vi "Test Base Main.vi"() -> ()   [LabVIEW 2013]
doc: "This Continuous Measurement sample project is based on the Queued Message Handler template.\n\nThe Event Handling Loop generates messages based on user interface actions.\n\nThe Message Handling Loop processes messages generated by the Event Handling Loop, or by other messages. There are also Acquisition and Logging message handling loop subVIs, and a chart updating loop."
uses:
  Settings/Settings.ctl
  Acquisition/Hardware Configuration.ctl
  Acquisition/Signal Type.ctl
  Logging/Logging Configuration.ctl
  controls/UI Data.ctl
  controls/UI State.ctl
  <vilib>/Utility/error.llb/DialogType.ctl
  support/Message Queue/Message Cluster.ctl
  support/Message Queue/Enqueue Message (Single).vi
  <vilib>/Utility/error.llb/Error Cluster From Error Code.vi
  <vilib>/ErrorRing/Error Ring.xnode
  Acquisition/Acquisition.lvlib
  Logging/Logging.lvlib
  Settings/Settings.lvlib
  support/User Event - Stop/User Event - Stop.lvlib
  support/Message Queue/Message Queue.lvlib
  support/Message Queue/Enqueue Message (MultiLine String w Array).vi
panel:
  in  "Test Logging Error Handler":bool
  in  "Test Acquisition Error Handler":bool
  out "Data":waveform(dbl)[](graph)
  in  "Settings":bool
  in  "Start":bool
  in  "Stop":bool
  out "Status":string
  in  "Exit":bool
  # "Continuous Measurement Data Logger"
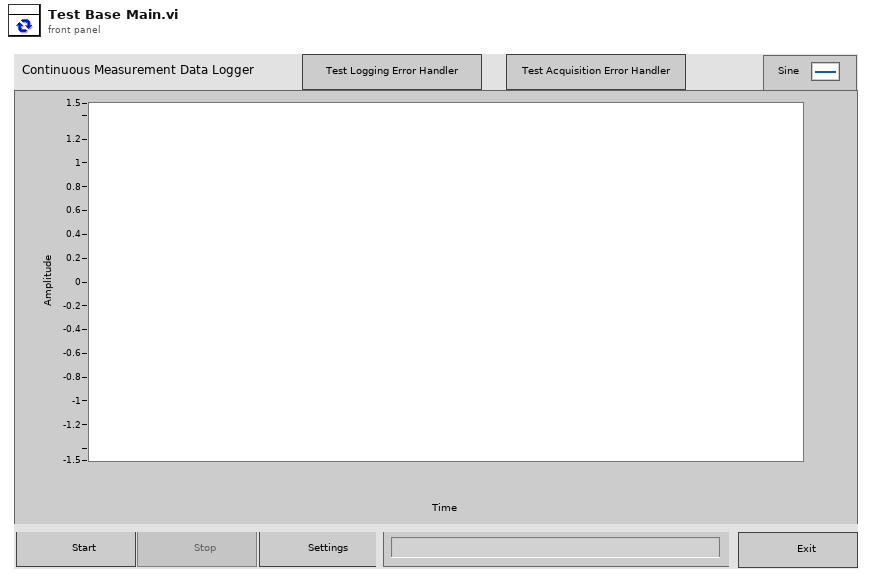
[diagram p1: front panel]
types:
  T1 = cluster{"Macro:Initialize":string, "Macro:Exit":string, "Core":cluster{"Current VI Reference":refnum<vi>, "Close Panel on Exit?":bool}}
  T2 = typedef "UI State.ctl" = enum16{"Idle", "Acquiring and Logging", "Waiting for Exit", "Waiting for Exit (Acq Stopped)", "Waiting for Exit (Log Stopped)", "Waiting for Stop", "Waiting for Stop (Acq Stopped)", "Waiting for Stop (Log Stopped)"}
  T3 = typedef "UI Data.ctl" = cluster{"Start Ref":refnum<vi>, "Stop Ref":refnum<vi>, "Settings Ref":refnum<vi>, "Exit Ref":refnum<vi>, "Status Ref":refnum<vi>, "Data Ref":refnum<vi>}
  T4 = typedef "Settings.lvlib/Settings.ctl" = cluster{"Hardware Configuration":T5, "Logging Configuration":T7}
  T5 = typedef "Acquisition.lvlib/Hardware Configuration.ctl" = cluster{"HW Refnum <Replace Me>":string, "Signal Type <Replace Me>":T6}
  T6 = typedef "Acquisition.lvlib/Signal Type.ctl" = enum16{"Sine Wave", "Square with Noise"}
  T7 = typedef "Logging.lvlib/Logging Configuration.ctl" = cluster{"Log File Base Path":path, "TDMS File Reference":refnum<k34>}
  T8 = typedef "Message Queue.lvlib/All Message Queues.ctl" = cluster{"UI":refnum<queue>, "Acquisition":refnum<queue>, "Logging":refnum<queue>}
  T9 = enum32{"invalid app kind", "Development System", "Run Time System", "Student Edition", "Embedded LabVIEW", "Evaluation", "Custom"}
  T10 = typedef "Message Queue.lvlib/Message Cluster.ctl" = cluster{"Message":string, "Message Data":variant}
  T11 = enum32{"Invalid", "Standard", "Closed", "Hidden", "Minimized", "Maximized"}
  T12 = typedef "DialogType.ctl" = u16
  T13 = cluster{"element":T10, "error constant":errorcluster}
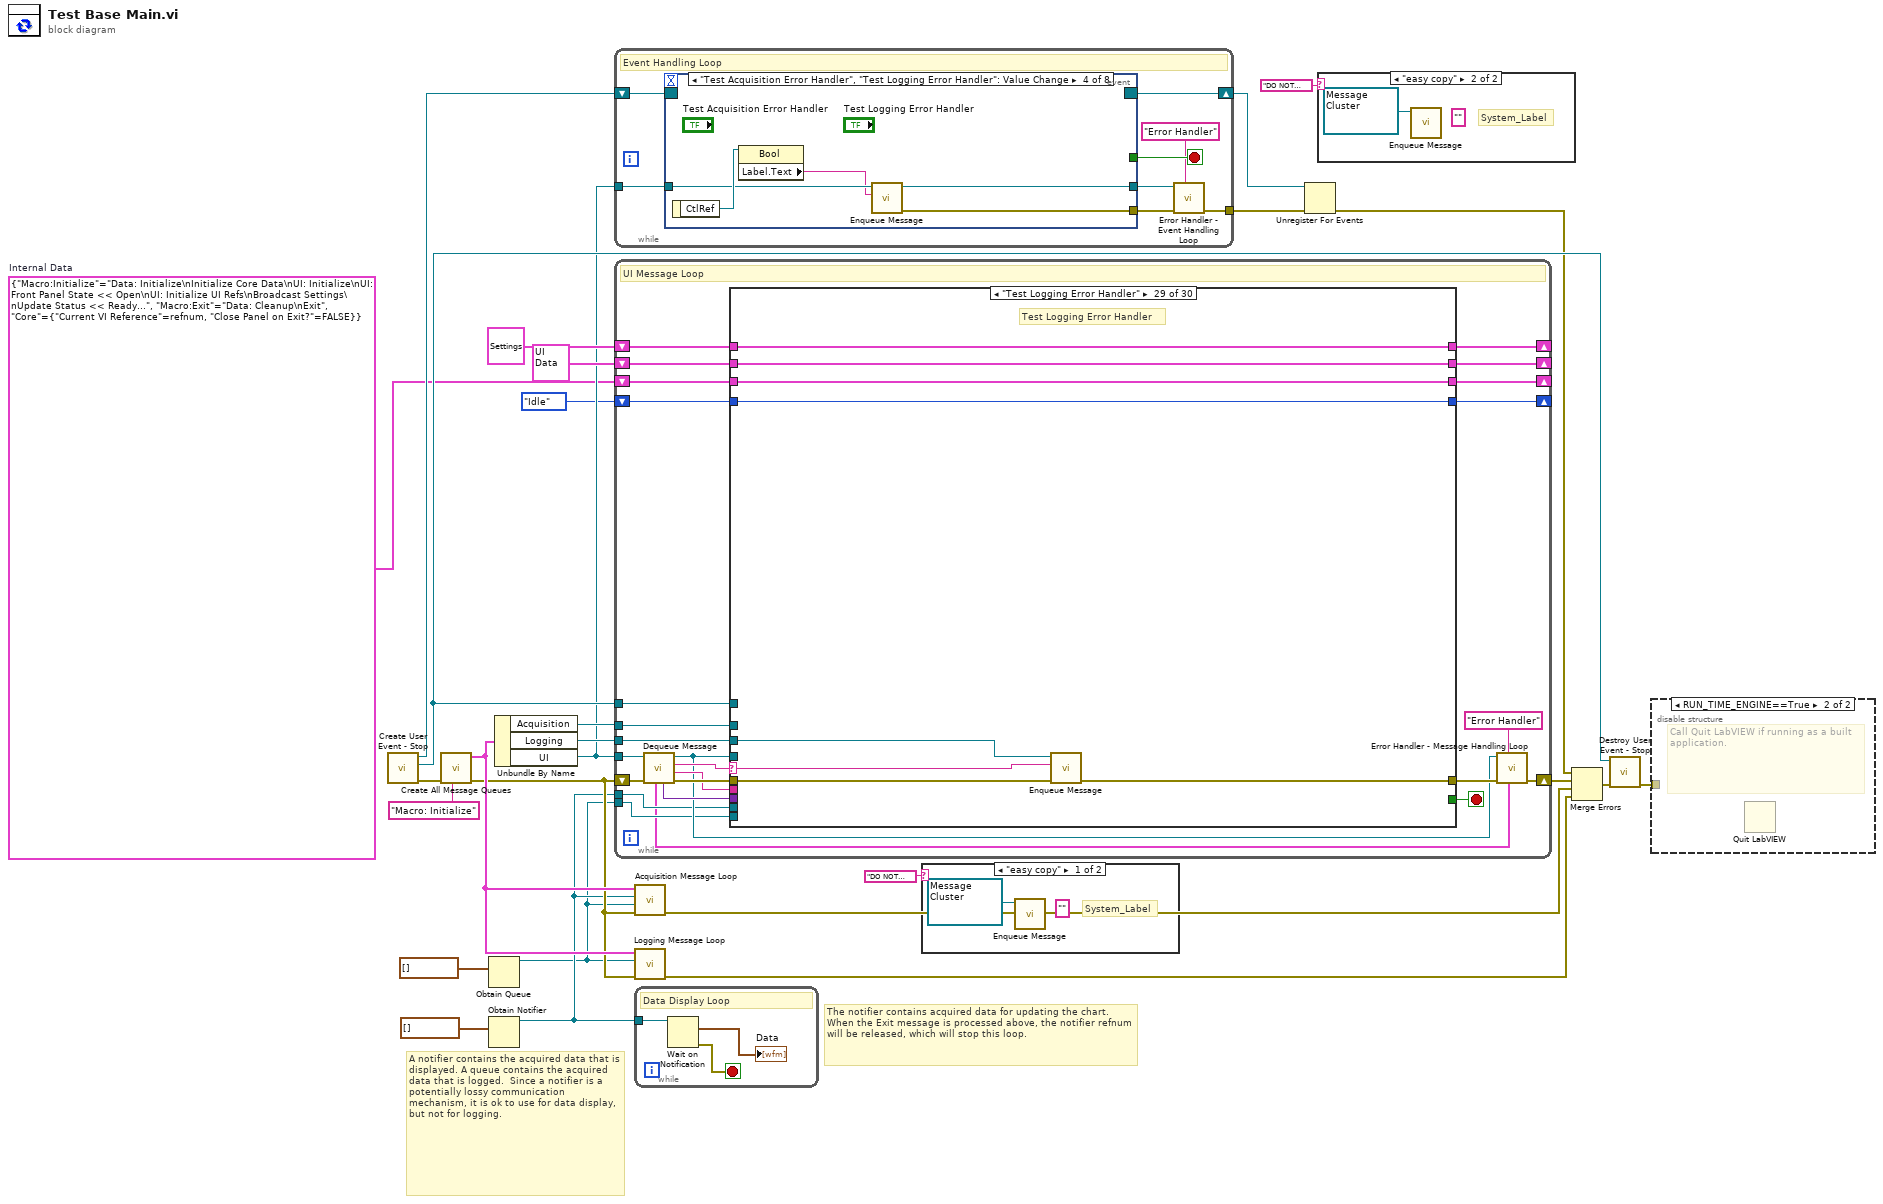
[diagram p0: block diagram]
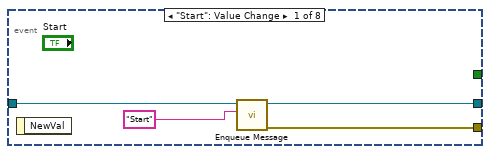
[diagram p5: hidden frame]
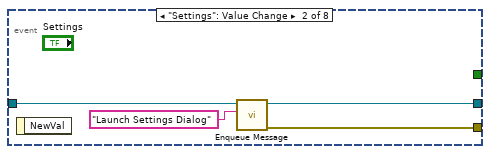
[diagram p6: hidden frame]
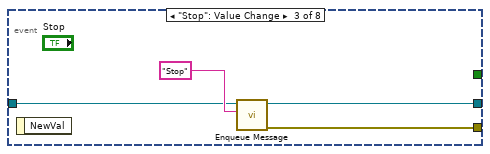
[diagram p7: hidden frame]
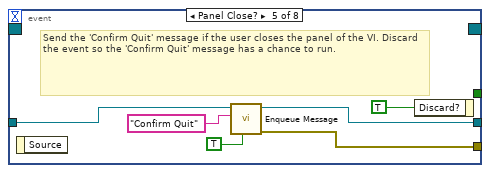
[diagram p8: hidden frame]
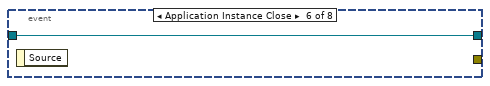
[diagram p9: hidden frame]
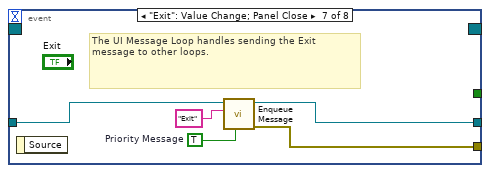
[diagram p10: hidden frame]
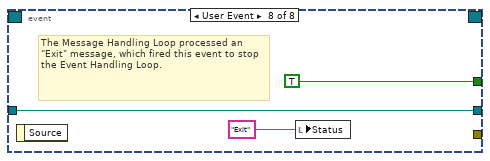
[diagram p11: hidden frame]
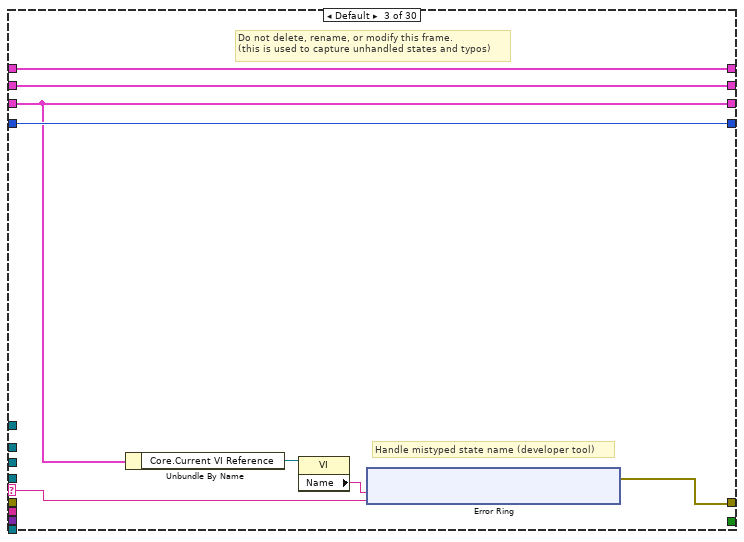
[diagram p14: hidden frame]
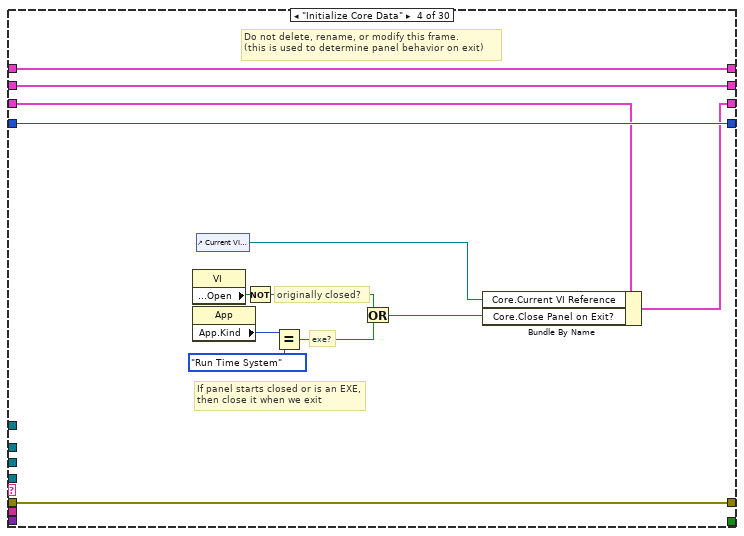
[diagram p15: hidden frame]
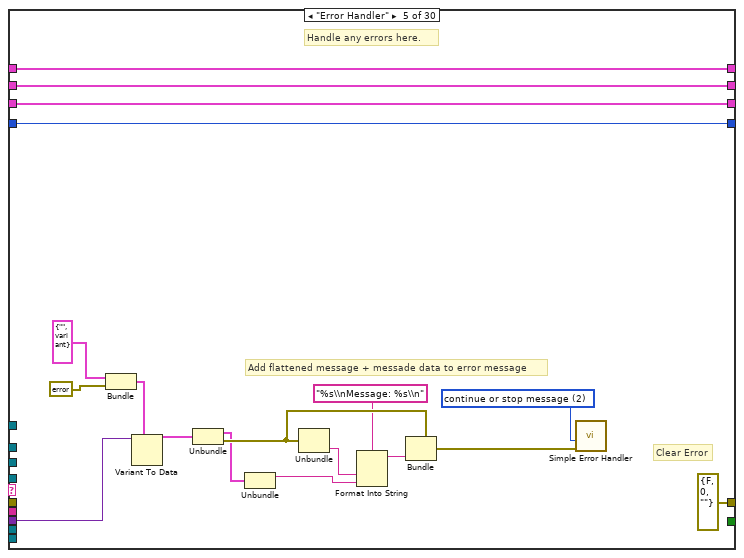
[diagram p16: hidden frame]
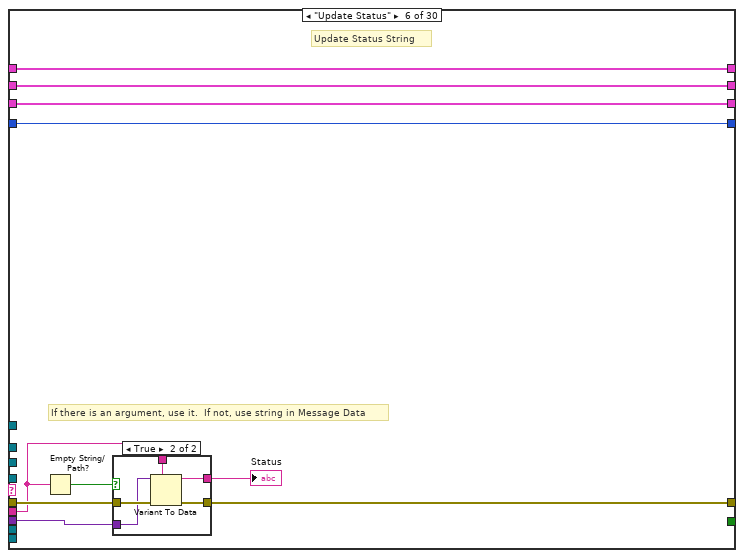
[diagram p17: hidden frame]
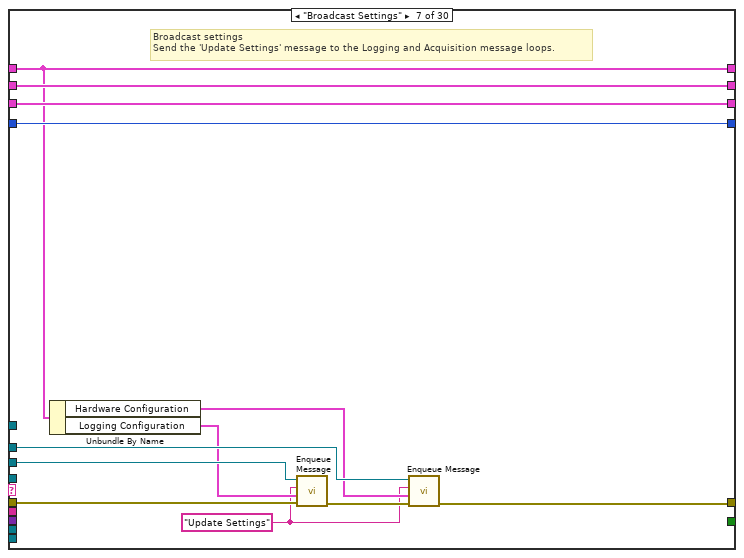
[diagram p19: hidden frame]
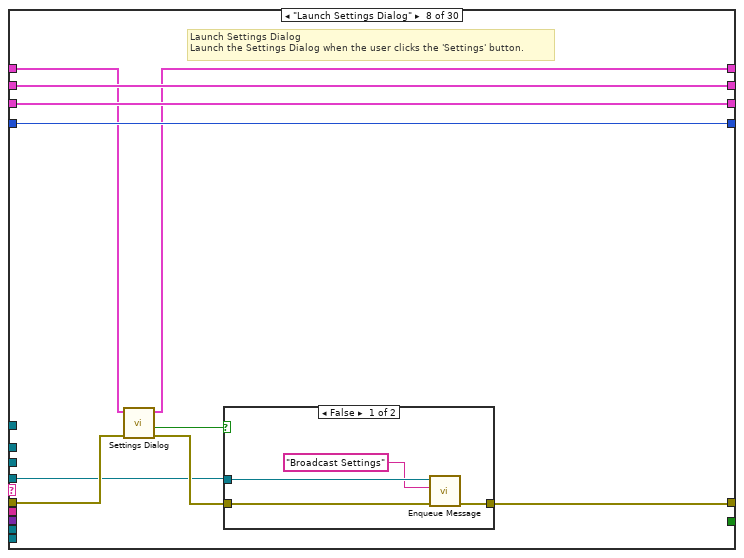
[diagram p20: hidden frame]
diagram:
  w4 = T1 {"Macro:Initialize"="Data: Initialize\nInitialize Core Data\nUI: Initialize\nUI: Front Panel State << Open\nUI: Initialize UI Refs\nBroadcast Settings\nUpdate Status << Ready...", "Macro:Exit"="Data: Cleanup\nExit", "Core"={"Current VI Reference"=refnum, "Close Panel on Exit?"=FALSE}}  # Internal Data
  # "A notifier contains the acquired data that is displayed. A queue contains the acquired data that is logged.  Since a notifier is a potentially lossy communication mechanism, it is ok to use for data display, but not for logging."
  # "The notifier contains acquired data for updating the chart. When the Exit message is processed above, the notifier refnum will be released, which will stop this loop."
  n1 = call "Create User Event - Stop.vi"() -> ("error out"=w22:errorcluster, "User Event - Stop"=w24:refnum<user-event>, "Stop Event Registration Refnum"=w25:refnum<event-registration>)  [unwired: 9 in]
  n2 = call "Create All Message Queues.vi"("Message"="Macro: Initialize", "error in (no error)"=w22) -> ("error out"=w19:errorcluster, "Message Queues out"=w21:T8)  [unwired: 8 in]
  n3 = Obtain Queue(element data type=waveform(dbl)[] []) -> (queue out=w8:refnum<queue>)  [unwired: 4 in, 2 out]
  n4 = Obtain Notifier(notification data type=waveform(dbl)[] []) -> (notifier out=w10:refnum<notifier>)  [unwired: 3 in, 2 out]
  n5 = Unbundle By Name(w21) -> ("Acquisition"=w14:refnum<queue>, "Logging"=w13:refnum<queue>, "UI"=w12:refnum<queue>)
  n6 = while {
    tunnel: w12 -> [w34]
    tunnel: [w31] -> w26
    shift-right: [w33] -> w16
    shift-left: w25 -> [w35]
    stop <- w32 stop-if-true
    # "Event Handling Loop"
    n7 = event shown="[3] \"Test Acquisition Error Handler\", \"Test Logging Error Handler\": Value Change" {
      selector: w35 -> [_ _ _ _ _ _ _ _]
      dyn-events: [_ _ _ _ _ _ _ _] -> w33
      timeout: _ -> [_ _ _ _ _ _ _ _]
      tunnel: [_ _ _ _ _ _ _ TRUE ("Discard?")] -> w32
      tunnel: w34 -> [w39 w41 w46 w51 w56 w59 w61 w65]
      tunnel: [w37 w43 w45 w49 w54 _ w64 _] -> w30
      tunnel: [w36 w40 w44 w50 w55 w59 w60 w65] -> w29
      event "Start": Value Change {
        n8 = event-data() -> ()  [unwired: 1 in, 1 out]
        n9 = call-poly "Enqueue Message.vi"("Message"="Start", "Message Queue"=w39) -> ("error out"=w37:errorcluster, "dup Message Queue"=w36:refnum<queue>)  [unwired: 8 in]
      }
      event "Settings": Value Change {
        n10 = event-data() -> ()  [unwired: 1 in, 1 out]
        n11 = call-poly "Enqueue Message.vi"("Message"="Launch Settings Dialog", "Message Queue"=w41) -> ("error out"=w43:errorcluster, "dup Message Queue"=w40:refnum<queue>)  [unwired: 8 in]
      }
      event "Stop": Value Change {
        n12 = event-data() -> ()  [unwired: 1 in, 1 out]
        n13 = call-poly "Enqueue Message.vi"("Message"="Stop", "Message Queue"=w46) -> ("error out"=w45:errorcluster, "dup Message Queue"=w44:refnum<queue>)  [unwired: 8 in]
      }
      event "Test Acquisition Error Handler", "Test Logging Error Handler": Value Change {
        n14 = event-data() -> ("CtlRef"=w52:refnum<vi>)  [unwired: 1 in]
        n15 = property class="Bool"(reference=w52) -> ("Label.Text"=w48:string)  [unwired: 1 in, 2 out]
        n16 = call-poly "Enqueue Message.vi"("Message"=w48, "Message Queue"=w51) -> ("error out"=w49:errorcluster, "dup Message Queue"=w50:refnum<queue>)  [unwired: 8 in]
      }
      event Panel Close? {
        # "Send the 'Confirm Quit' message if the user closes the panel of the VI. Discard the event so the 'Confirm Quit' message has a chance to run."
        n17 = event-data() -> ()  [unwired: 1 in, 1 out]
        n18 = call-poly "Enqueue Message.vi"("Priority Message? (F)"=TRUE, "Message"="Confirm Quit", "Message Queue"=w56) -> ("error out"=w54:errorcluster, "dup Message Queue"=w55:refnum<queue>)  [unwired: 7 in]
        n19 = event-data("Discard?"=TRUE) -> ()  [unwired: 1 in, 1 out]
      }
      event Application Instance Close {
        n20 = event-data() -> ()  [unwired: 1 in, 1 out]
      }
      event "Exit": Value Change; Panel Close {
        w62 = TRUE  # Priority Message
        # "The UI Message Loop handles sending the Exit message to other loops."
        n21 = event-data() -> ()  [unwired: 1 in, 1 out]
        n22 = call-poly "Enqueue Message.vi"("Priority Message? (F)"=w62, "Message"="Exit", "Message Queue"=w61) -> ("error out"=w64:errorcluster, "dup Message Queue"=w60:refnum<queue>)  [unwired: 7 in]
      }
      event User Event {
        # "The Message Handling Loop processed an \"Exit\" message, which fired this event to stop the Event Handling Loop."
        n23 = event-data() -> ()  [unwired: 1 in, 1 out]
        n24 = local write "Status"("Exit" ("Exit String")) -> ()
      }
    }
    n25 = call "Error Handler - Event Handling Loop.vi"("Error Handler Message"="Error Handler" ("Message"), "error in (no error)"=w30, "Message Queue"=w29) -> ("dup error in"=w31:errorcluster)  [unwired: 7 in, 1 out]
  }
  n26 = while {
    tunnel: w12 -> [w91]
    tunnel: w24 -> [w87]
    shift-right: [w90] -> w27
    shift-left: w19 -> [w92]
    shift-right: [w78] -> _
    shift-left: T4 {"Hardware Configuration"={"HW Refnum <Replace Me>"="", "Signal Type <Replace Me>"=enum."Sine Wave"}, "Logging Configuration"={"Log File Base Path"=path "", "TDMS File Reference"=refnum}} ("Settings") -> [w80]
    shift-right: [w77] -> _
    shift-left: T3 {"Start Ref"=refnum, "Stop Ref"=refnum, "Settings Ref"=refnum, "Exit Ref"=refnum, "Status Ref"=refnum, "Data Ref"=refnum} ("Measurement UI Controls") -> [w79]
    tunnel: w14 -> [w86]
    tunnel: w13 -> [w85]
    tunnel: w10 -> [w70]
    tunnel: w8 -> [w69]
    shift-right: [w84] -> _
    shift-left: UI_State."Idle" ("UI State") -> [w83]
    shift-right: [w73] -> _
    shift-left: w4 -> [w74]
    stop <- w82 stop-if-true
    # "UI Message Loop"
    n27 = call "Dequeue Message.vi"("error in (no error)"=w92, "Message Queue"=w91) -> ("error out"=w89:errorcluster, "Argument"=w76:string, "Message"=w88:string, "dup Message Queue"=w72:refnum<queue>, "Message Data"=w75:variant, "element"=w68:T10)  [unwired: 4 in]
    n28 = case shown="\"Test Logging Error Handler\"" w88 {
      selector: w88 -> [_ _ w104 _ _ _ _ _ _ _ _ _ _ _ _ _ _ _ _ _ w346 _ _ _ _ _ _ w471 w480 _]
      tunnel: w79 -> [w96 w100 w109 w123 w149 w158 w178 w188 w201 w238 w243 w252 w255 w262 w267 w279 w292 w303 w333 w342 w361 w367 w388 w408 w418 w444 w467 w476 w484 w488]
      tunnel: w76 -> [_ _ _ _ _ w151 _ _ _ _ _ _ _ _ _ _ w293 w304 _ _ _ _ _ _ _ _ _ _ _ _]
      tunnel: w80 -> [w95 w101 w110 w121 w147 w159 w171 w185 w195 w240 w244 w250 w256 w263 w269 w289 w296 w306 w334 w343 w359 w368 w390 w410 w420 w446 w468 w477 w485 w489]
      tunnel: [w97 w102 w103 w131 errorcluster {"status"=FALSE, "code"=0, "source"=""} ("error out") w153 w167 w179 w194 w230 w245 w248 w257 w264 w268 w288 w294 w307 w335 w338 w348 w369 w371 w391 w415 w439 w469 w470 w479 w490] -> w81
      tunnel: w89 -> [w97 w102 _ w131 _ w155 w175 w183 w198 w228 w245 w249 w258 w264 w268 w288 w295 w308 w335 w340 w358 w369 w378 w393 w416 w440 w469 w473 w481 w490]
      tunnel: [w96 w100 w109 w123 w149 w158 w178 w188 w201 w238 w243 w252 w255 w262 w267 w270 w292 w303 w333 w342 w361 w367 w388 w408 w418 w444 w467 w476 w484 w488] -> w77
      tunnel: [_ _ _ _ _ _ _ _ _ TRUE _ _ _ _ _ _ _ _ _ _ _ _ _ _ _ _ _ _ _ _] -> w82
      tunnel: [w95 w101 w110 w121 w147 w159 w171 w184 w195 w240 w244 w247 w256 w263 w269 w289 w296 w306 w334 w343 w359 w368 w390 w410 w420 w446 w468 w477 w485 w489] -> w78
      tunnel: w87 -> [_ _ _ _ _ _ _ _ _ w229 _ _ _ _ _ _ _ _ _ _ _ _ _ _ _ _ _ _ _ _]
      tunnel: w86 -> [_ _ _ _ _ _ w172 _ _ w227 _ _ _ _ _ _ _ _ _ _ w344 _ w373 w398 _ _ _ w472 _ _]
      tunnel: w85 -> [_ _ _ _ _ _ w174 _ _ w226 _ _ _ _ _ _ _ _ _ _ w345 _ w375 w399 _ _ _ _ w478 _]
      tunnel: [w94 w99 w108 w122 w148 w157 w177 w187 w196 UI_State."Idle" ("UI State") w242 w251 w254 w261 w266 w287 w291 w302 w332 w341 w360 w366 UI_State."Acquiring and Logging" ("UI State") w394 w414 w442 w466 w475 w483 w487] -> w84
      tunnel: w83 -> [w94 w99 w108 w122 w148 w157 w177 w187 w197 _ w242 w251 w254 w261 w266 w287 w291 w302 w332 w341 w360 w366 _ w395 w413 w443 w466 w475 w483 w487]
      tunnel: w75 -> [_ _ _ _ w132 w154 _ _ _ _ _ _ _ _ _ _ _ _ _ _ _ _ _ _ _ _ _ _ _ _]
      tunnel: w74 -> [w93 w98 w106 w120 w146 w156 w176 w186 w200 w237 w241 w246 w253 w260 w265 w286 w290 w301 w331 w336 w352 w365 w389 w409 w419 w445 w465 w474 w482 w486]
      tunnel: [w93 w98 w106 w119 w146 w156 w176 w186 w200 w237 w241 w246 w253 w260 w265 w286 w290 w301 w331 w336 w352 w365 w389 w409 w419 w445 w465 w474 w482 w486] -> w73
      tunnel: w72 -> [_ _ _ _ _ _ _ w180 w199 w225 _ _ _ _ _ _ _ _ _ w339 w357 _ w377 _ w417 w441 _ _ _ _]
      tunnel: w70 -> [_ _ _ _ _ _ _ _ _ w224 _ _ _ _ _ _ _ _ _ _ _ _ _ _ _ _ _ _ _ _]
      tunnel: w69 -> [_ _ _ _ _ _ _ _ _ w223 _ _ _ _ _ _ _ _ _ _ _ _ _ _ _ _ _ _ _ _]
      frame "", "Idle" {
        # "Executes when the state queue is empty\nAlso commented out messages"
      }
      frame "---------- Core ----------" {
        # "Do not put any code in this frame.\n(it is a separator no-op)"
      }
      frame Default {
        # "Handle mistyped state name (developer tool)"
        # "Do not delete, rename, or modify this frame.\n(this is used to capture unhandled states and typos)"
        n29 = Unbundle By Name(w106) -> ("Core.Current VI Reference"=w105:refnum<vi>)
        n30 = property class="VI"(reference=w105) -> ("Name"=w107:string)  [unwired: 1 in, 2 out]
        n31 = xnode "Error Ring"("parameter 0"=w107, "parameter 1"=w104) -> ("error out"=w103:errorcluster)
      }
      frame "Initialize Core Data" {
        # "Do not delete, rename, or modify this frame.\n(this is used to determine panel behavior on exit)"
        # "originally closed?"
        # "exe?"
        # "If panel starts closed or is an EXE, then close it when we exit"
        n32 = property class="VI"() -> ("Front Panel.Open"=w130:bool)  [unwired: 2 in, 2 out]
        n33 = property class="App"() -> ("App.Kind"=w129:T9)  [unwired: 2 in, 2 out]
        n34 = control-ref of="Current VI Reference"() -> (w124:refnum<vi>)
        n35 = Not(x=w130) -> (.not. x?=w127:bool)
        n36 = Equal?(x=w129, y=T9."Run Time System" ("Application:Kind")) -> (x = y?=w126:bool)
        n37 = Or(x=w127, y=w126) -> (x .or. y?=w125:bool)
        n38 = Bundle By Name(cluster=w120, "Core.Current VI Reference"=w124, "Core.Close Panel on Exit?"=w125) -> (w119:T1)
      }
      frame "Error Handler" {
        w144 = T12 2 items=["no dialog", "OK message", "continue or stop message", "OK message + warnings", "continue/stop + warnings"] ("type of dialog (OK msg:1)")
        # "Add flattened message + messade data to error message"
        # "Clear Error"
        # "Handle any errors here."
        n39 = Bundle("element"=T10 {"Message"="", "Message Data"=variant}, "error constant"=errorcluster {"status"=FALSE, "code"=0, "source"=""}) -> (w141:T13)  [unwired: 1 in]
        n40 = Variant To Data(type=w141, Variant=w132) -> (data=w140:T13)  [unwired: 1 in, 1 out]
        n41 = Unbundle(w140) -> ("element"=w137:T10, "error constant"=w139:errorcluster)
        n42 = Unbundle(w137) -> ("Message"=w135:string)  [unwired: 1 out]
        n43 = Unbundle(w139) -> ("source"=w134:string)  [unwired: 2 out]
        n44 = Format Into String(format string="%s\\nMessage: %s\\n", w134, w135) -> (resulting string=w136:string)  [unwired: 2 in, 1 out]
        n45 = Bundle(cluster=w139, "source"=w136) -> (w138:errorcluster)  [unwired: 2 in]
        n46 = call <vilib>:"Simple Error Handler.vi"("type of dialog (OK msg:1)"=w144, "error in (no error)"=w138) -> ()  [unwired: 3 in, 5 out]
      }
      frame "Update Status" {
        # "If there is an argument, use it.  If not, use string in Message Data"
        # "Update Status String"
        n47 = Empty String/Path?(string/path=w151) -> (empty?=w152:bool)
        n48 = case shown="True" w152 {
          tunnel: w155 -> [w160 w166]
          tunnel: w154 -> [_ w165]
          tunnel: w151 -> [w161 w164]
          tunnel: [w160 w163] -> w153
          tunnel: [w161 w162] -> w150
          frame False {
          }
          frame True {
            n49 = Variant To Data(error in=w166, type=w164, Variant=w165) -> (data=w162:string, error out=w163:errorcluster)
          }
        }
        "Status" <- w150
      }
      frame "Broadcast Settings" {
        w168 = "Update Settings" ("Message")
        # "Broadcast settings\nSend the 'Update Settings' message to the Logging and Acquisition message loops."
        n50 = Unbundle By Name(w171) -> ("Hardware Configuration"=w169:T5, "Logging Configuration"=w170:T7)
        n51 = call-poly "Enqueue Message.vi"("error in (no error)"=w175, "Message Data"=w170, "Message"=w168, "Message Queue"=w174) -> ("error out"=w173:errorcluster)  [unwired: 6 in, 1 out]
        n52 = call-poly "Enqueue Message.vi"("error in (no error)"=w173, "Message Data"=w169, "Message"=w168, "Message Queue"=w172) -> ("error out"=w167:errorcluster)  [unwired: 6 in, 1 out]
      }
      frame "Launch Settings Dialog" {
        # "Launch Settings Dialog\nLaunch the Settings Dialog when the user clicks the 'Settings' button."
        n53 = call "Settings Dialog.vi"("error in (no error)"=w183, "Settings in"=w185) -> ("error out"=w181:errorcluster, "Cancelled?"=w182:bool, "Settings out"=w184:T4)  [unwired: 6 in, 1 out]
        n54 = case shown="False" w182 {
          tunnel: w180 -> [w192 _]
          tunnel: w181 -> [w191 w193]
          tunnel: [w190 w193] -> w179
          frame False {
            n55 = call-poly "Enqueue Message.vi"("error in (no error)"=w191, "Message"="Broadcast Settings", "Message Queue"=w192) -> ("error out"=w190:errorcluster)  [unwired: 7 in, 1 out]
          }
          frame True {
          }
        }
      }
      frame "Confirm Quit" {
        # "Confirm Quit\nMessage that can confirm whether or not the user wants to exit the application."
        n56 = case shown="\"Acquiring and Logging\"" w197 {
          tunnel: w199 -> [w207 w211]
          tunnel: w198 -> [w206 w210]
          tunnel: [w205 w209] -> w194
          tunnel: [UI_State."Idle" ("UI State") w208] -> w196
          frame Default {
            # "If 'Confirm Quit' comes in while the system is idle, there is no need for a confirmation message."
            n57 = call-poly "Enqueue Message.vi"("Priority Message? (F)"=TRUE, "error in (no error)"=w206, "Message"="Exit", "Message Queue"=w207) -> ("error out"=w205:errorcluster)  [unwired: 6 in, 1 out]
          }
          frame "Acquiring and Logging" {
            n58 = Two Button Dialog(message="Are you sure you want to quit while the acquisition is running?" ("Confirm Quit Message"), 1:"No" ("No"), 2:"Yes" ("Yes")) -> (T button?=w212:bool)
            n59 = case shown="True" w212 {
              tunnel: w211 -> [_ w221]
              tunnel: w210 -> [w217 w222]
              tunnel: [w217 w220] -> w209
              tunnel: [UI_State."Acquiring and Logging" ("UI State") UI_State."Waiting for Exit" ("UI State")] -> w208
              frame False {
                # "User did not want to quit."
              }
              frame True {
                n60 = call-poly "Enqueue Message.vi"("error in (no error)"=w222, "Message"="Stop", "Message Queue"=w221) -> ("error out"=w220:errorcluster)  [unwired: 7 in, 1 out]
              }
            }
          }
        }
      }
      frame "Exit" {
        w235 = "Exit" ("Message")
        # "Don't check the error outs. The acquisition and logging queues may have already been released."
        # "Close references owned by the Main VI."
        # "Stop the VI"
        # "Exit\nFire the User Event to stop the Event Handling Loop.  Also send Exit messages to the Acquisition and Logging loops."
        n61 = Release Queue(queue=w225, error in (no error)=w228) -> (error out=w234:errorcluster)  [unwired: 1 in, 2 out]
        n62 = call "Fire User Event - Stop.vi"("User Event - Stop"=w229) -> ("error out"=w236:errorcluster)  [unwired: 10 in]
        n63 = Release Notifier(notifier=w224, error in (no error)=w234) -> (error out=w233:errorcluster)  [unwired: 1 in, 2 out]
        n64 = Release Queue(queue=w223, error in (no error)=w233) -> (error out=w232:errorcluster)  [unwired: 1 in, 2 out]
        n65 = call-poly "Enqueue Message.vi"("Message"=w235, "Message Queue"=w227) -> ()  [unwired: 8 in, 2 out]
        n66 = call-poly "Enqueue Message.vi"("Message"=w235, "Message Queue"=w226) -> ()  [unwired: 8 in, 2 out]
        n67 = Merge Errors(w236, w232) -> (w230:errorcluster)
      }
      frame "---------- Data ----------" {
        # "Do not put any code in this frame.\n(It is a separator no-op. You can make a copy of this frame to create a new Data frame)"
      }
      frame "Data: Initialize" {
        # "nothing right now"
        # "Initialize the shift-register data, here.\n(data names are defined by what you wire into the bundle function)"
        n68 = call "Load Settings from XML.vi"("error in (no error)"=w249, "Settings in"=w250) -> ("error out"=w248:errorcluster, "Settings out"=w247:T4)  [unwired: 8 in]
      }
      frame "Data: Cleanup" {
        # "Cleanup any data and references, here.\n(this is called automatically, by the Macro: Exit)"
        n69 = Unbundle By Name(w253) -> ("Core.Current VI Reference"=w259:refnum<vi>)
        n70 = Close Reference(reference=w259, error in (no error)=w258) -> (error out=w257:errorcluster)
      }
      frame "---------- UI ----------" {
        # "Do not put any code in this frame.\n(It is a separator no-op. You can make a copy of this frame to create a new UI frame)"
      }
      frame "UI: Initialize" {
        # "Initialize the User Interface, here.\n(this is called automatically, by the Macro: Init)"
      }
      frame "UI: Initialize UI Refs" {
        # "Enable: Start, Exit, Settings\nDisable: Stop"
        # "Package and Init UI Refs as Required"
        n71 = control-ref of="Data"() -> (w280:refnum<vi>)
        n72 = control-ref of="Start"() -> (w285:refnum<vi>)
        n73 = control-ref of="Stop"() -> (w283:refnum<vi>)
        n74 = control-ref of="Settings"() -> (w284:refnum<vi>)
        n75 = control-ref of="Exit"() -> (w282:refnum<vi>)
        n76 = control-ref of="Status"() -> (w281:refnum<vi>)
        n77 = Bundle By Name(cluster=w279, "Start Ref"=w285, "Stop Ref"=w283, "Settings Ref"=w284, "Exit Ref"=w282, "Status Ref"=w281, "Data Ref"=w280) -> (w270:T3)
        n78 = Unbundle By Name(w270) -> ("Stop Ref"=w278:refnum<vi>, "Start Ref"=w275:refnum<vi>, "Exit Ref"=w274:refnum<vi>, "Settings Ref"=w273:refnum<vi>)
        n79 = Build Array(w278) -> (w277:refnum<vi>[])
        n80 = Build Array(w275, w274, w273) -> (w272:refnum<vi>[])
        n81 = call "Set Enable State on Multiple Controls.vi"("Enable?"=TRUE, "Controls"=w272) -> ()  [unwired: 10 in]
        n82 = call "Set Enable State on Multiple Controls.vi"("Enable?"=FALSE, "Controls"=w277) -> ()  [unwired: 10 in]
      }
      frame "UI: Cursor Set" {
        # "Argument"
        # "Set and Unset Cursor Busy.\n(Usage: \"UI: Cursor Set >> Busy|Idle\")"
        n83 = case shown="\"Idle\", Default" w293 {
          tunnel: w295 -> [w298 w300]
          tunnel: [w297 w299] -> w294
          frame "Idle", Default {
            n84 = call <vilib>:"Unset Busy.vi"("error in (no error)"=w298) -> ("error out"=w297:errorcluster)  [unwired: 10 in]
          }
          frame "Busy" {
            n85 = call <vilib>:"Set Busy.vi"("error in (no error)"=w300) -> ("error out"=w299:errorcluster)  [unwired: 9 in, 1 out]
          }
        }
      }
      frame "UI: Front Panel State" {
        # "Argument"
        # "Set Front Panel Open or Closed\n(Usage: \"UI: Front Panel State >> Open|Close\")"
        n86 = Unbundle By Name(w301) -> ("Core.Current VI Reference"=w305:refnum<vi>)
        n87 = case shown="\"Open\", Default" w304 {
          tunnel: w308 -> [w312 w325]
          tunnel: [w314 w326] -> w307
          tunnel: w305 -> [w313 w323]
          frame "Open", Default {
            n88 = property class="VI"(reference=w313, error in=w312) -> (reference out=w310:refnum<vi>, error out=w311:errorcluster, "Front Panel.Open"=w309:bool)
            n89 = case shown="True" w309 {
              tunnel: [w317 w320] -> w314
              tunnel: w311 -> [w316 w320]
              tunnel: w310 -> [w315 _]
              frame False {
                n90 = invoke class="VI" method="FP.Open"(reference=w315, error in=w316, "Activate"=TRUE, "State"=T11."Standard") -> (error out=w317:errorcluster)  [unwired: 1 in, 4 out]
              }
              frame True {
              }
            }
          }
          frame "Close" {
            n91 = property class="VI"(reference=w323, error in=w325) -> (reference out=w322:refnum<vi>, error out=w324:errorcluster, "Front Panel.Open"=w321:bool)
            n92 = case shown="True" w321 {
              tunnel: [w327 w330] -> w326
              tunnel: w324 -> [w327 w329]
              tunnel: w322 -> [_ w328]
              frame False {
              }
              frame True {
                n93 = invoke class="VI" method="FP.Close"(reference=w328, error in=w329) -> (error out=w330:errorcluster)  [unwired: 1 in, 2 out]
              }
            }
          }
        }
      }
      frame "---------- Macro ----------" {
        # "Do not put any code in this frame.\n(It is a separator no-op. You can make a copy of this frame to create a new Macro frame)"
      }
      frame "Macro: Initialize" {
        # "Initialization Macro\n(This is called once, when the VI starts)"
        n94 = Unbundle By Name(w336) -> ("Macro:Initialize"=w337:string)
        n95 = call-poly "Enqueue Message.vi"("error in (no error)"=w340, "Message"=w337, "Message Queue"=w339) -> ("error out"=w338:errorcluster)  [unwired: 7 in, 1 out]
      }
      frame "Macro: Exit" {
        w347 = FALSE ("Priority Message? (F)")
        # "Exit Macro\n(This is called once, when the VI exits)"
        n96 = Unbundle By Name(w352) -> ("Core.Close Panel on Exit?"=w364:bool)
        n97 = Unbundle By Name(w352) -> ("Macro:Exit"=w351:string)
        n98 = Select(t="UI: Front Panel State >> Close", s=w364, f="") -> (s? t:f=w356:string)
        n99 = call-poly "Enqueue Message.vi"("Priority Message? (F)"=TRUE, "error in (no error)"=w358, "Message"=w356, "Message Queue"=w357) -> ("error out"=w353:errorcluster, "dup Message Queue"=w354:refnum<queue>)  [unwired: 6 in]
        n100 = call-poly "Enqueue Message.vi"("Priority Message? (F)"=w347, "error in (no error)"=w353, "Message"=w351, "Message Queue"=w354) -> ("error out"=w350:errorcluster)  [unwired: 6 in, 1 out]
        n101 = call-poly "Enqueue Message.vi"("Priority Message? (F)"=w347, "error in (no error)"=w350, "Message"=w346, "Message Queue"=w345) -> ("error out"=w349:errorcluster)  [unwired: 6 in, 1 out]
        n102 = call-poly "Enqueue Message.vi"("Priority Message? (F)"=w347, "error in (no error)"=w349, "Message"=w346, "Message Queue"=w344) -> ("error out"=w348:errorcluster)  [unwired: 6 in, 1 out]
      }
      frame "---------- System ----------" {
        # "Template Separator\n(You can make a copy of, or modify, this frame)"
      }
      frame "Start" {
        w370 = "Start" ("Message")
        # "Message Acquisition and Logging loops to start."
        # "Enable: Stop\nDisable: Start, Exit, Settings"
        # "Start System\nStart - Enable/Disable buttons appropriately for an acquisition that has started, and update status display."
        n103 = Unbundle By Name(w388) -> ("Stop Ref"=w387:refnum<vi>, "Start Ref"=w384:refnum<vi>, "Exit Ref"=w383:refnum<vi>, "Settings Ref"=w382:refnum<vi>)
        n104 = call-poly "Enqueue Message.vi"("error in (no error)"=w378, "Message"="Update Status << Acquiring and Logging...", "Message Queue"=w377) -> ("error out"=w374:errorcluster)  [unwired: 7 in, 1 out]
        n105 = Build Array(w387) -> (w386:refnum<vi>[])
        n106 = Build Array(w384, w383, w382) -> (w381:refnum<vi>[])
        n107 = call-poly "Enqueue Message.vi"("error in (no error)"=w374, "Message"=w370, "Message Queue"=w375) -> ("error out"=w372:errorcluster)  [unwired: 7 in, 1 out]
        n108 = call "Set Enable State on Multiple Controls.vi"("Enable?"=FALSE, "Controls"=w381) -> ()  [unwired: 10 in]
        n109 = call "Set Enable State on Multiple Controls.vi"("Enable?"=TRUE, "Controls"=w386) -> ()  [unwired: 10 in]
        n110 = call-poly "Enqueue Message.vi"("error in (no error)"=w372, "Message"=w370, "Message Queue"=w373) -> ("error out"=w371:errorcluster)  [unwired: 7 in, 1 out]
      }
      frame "Stop" {
        w396 = "Stop" ("Message")
        # "Message Acquisition and Logging loops to stop"
        # "Enable: Start, Exit, Settings\nDisable: Stop"
        # "Stop System\nEnable/Disable buttons appropriately for an acquisition that has stopped, and update status display."
        n111 = Unbundle By Name(w408) -> ("Stop Ref"=w407:refnum<vi>, "Start Ref"=w404:refnum<vi>, "Exit Ref"=w403:refnum<vi>, "Settings Ref"=w402:refnum<vi>)
        n112 = Build Array(w407) -> (w406:refnum<vi>[])
        n113 = Build Array(w404, w403, w402) -> (w401:refnum<vi>[])
        n114 = call-poly "Enqueue Message.vi"("error in (no error)"=w393, "Message"=w396, "Message Queue"=w399) -> ("error out"=w397:errorcluster)  [unwired: 7 in, 1 out]
        n115 = call "Set Enable State on Multiple Controls.vi"("Enable?"=TRUE, "Controls"=w401) -> ()  [unwired: 10 in]
        n116 = call "Set Enable State on Multiple Controls.vi"("Enable?"=FALSE, "Controls"=w406) -> ()  [unwired: 10 in]
        n117 = call-poly "Enqueue Message.vi"("error in (no error)"=w397, "Message"=w396, "Message Queue"=w398) -> ("error out"=w392:errorcluster)  [unwired: 7 in, 1 out]
        n118 = Merge Errors(w392) -> (w391:errorcluster)
        n119 = case shown="Default" w395 {
          selector: w395 -> [w411 _]
          tunnel: [w411 UI_State."Waiting for Stop" ("UI State")] -> w394
          frame "Waiting for Exit" {
          }
          frame Default {
          }
        }
      }
      frame "Acquisition Stopped" {
        # "Logic for determining what action to take when the acquisition has stopped."
        n120 = case shown="\"Waiting for Stop (Log Stopped)\"" w413 {
          selector: w413 -> [w422 _ _ _ _]
          tunnel: w416 -> [w421 w424 w426 w432 w438]
          tunnel: w417 -> [_ _ _ w430 w435]
          tunnel: [w422 UI_State."Waiting for Exit (Acq Stopped)" ("UI State") UI_State."Waiting for Stop (Acq Stopped)" ("UI State") UI_State."Idle" ("UI State") UI_State."Idle" ("UI State")] -> w414
          tunnel: [w421 w424 w426 w431 w436] -> w415
          frame Default {
          }
          frame "Waiting for Exit", "Waiting for Exit (Acq Stopped)" {
          }
          frame "Waiting for Stop", "Waiting for Stop (Acq Stopped)" {
          }
          frame "Waiting for Exit (Log Stopped)" {
            # "If we are waiting to exit, and the logging has already stopped, then the \"Acquisition Stopped\" message indicates that it is time to exit."
            n121 = call-poly "Enqueue Message.vi"("Priority Message? (F)"=TRUE, "error in (no error)"=w432, "Message"="Exit", "Message Queue"=w430) -> ("error out"=w431:errorcluster)  [unwired: 6 in, 1 out]
          }
          frame "Waiting for Stop (Log Stopped)" {
            # "If we are waiting to stop, and the logging has already stopped, then the \"Acquisition Stopped\" message indicates that it is time to stop."
            n122 = call-poly "Enqueue Message.vi"("error in (no error)"=w438, "Message Data"="Ready..." ("Ready..."), "Message"="Update Status", "Message Queue"=w435) -> ("error out"=w436:errorcluster)  [unwired: 6 in, 1 out]
          }
        }
      }
      frame "Logging Stopped" {
        # "Logic for determining what action to take when the logging has stopped."
        n123 = case shown="\"Waiting for Stop (Acq Stopped)\"" w443 {
          selector: w443 -> [w448 _ _ _ _]
          tunnel: w440 -> [w447 w450 w452 w458 w461]
          tunnel: w441 -> [_ _ _ w456 w460]
          tunnel: [w448 UI_State."Waiting for Exit (Log Stopped)" ("UI State") UI_State."Waiting for Stop (Log Stopped)" ("UI State") UI_State."Idle" ("UI State") UI_State."Idle" ("UI State")] -> w442
          tunnel: [w447 w450 w452 w457 w459] -> w439
          frame Default {
          }
          frame "Waiting for Exit", "Waiting for Exit (Log Stopped)" {
          }
          frame "Waiting for Stop", "Waiting for Stop (Log Stopped)" {
          }
          frame "Waiting for Exit (Acq Stopped)" {
            # "If we are waiting to exit, and the acquisition has already stopped, then the \"Logging Stopped\" message indicates that it is time to exit."
            n124 = call-poly "Enqueue Message.vi"("Priority Message? (F)"=TRUE, "error in (no error)"=w458, "Message"="Exit", "Message Queue"=w456) -> ("error out"=w457:errorcluster)  [unwired: 6 in, 1 out]
          }
          frame "Waiting for Stop (Acq Stopped)" {
            # "If we are waiting to stop, and the acquisition has already stopped, then the \"Logging Stopped\" message indicates that it is time to stop."
            n125 = call-poly "Enqueue Message.vi"("error in (no error)"=w461, "Message Data"="Ready..." ("Ready..."), "Message"="Update Status", "Message Queue"=w460) -> ("error out"=w459:errorcluster)  [unwired: 6 in, 1 out]
          }
        }
      }
      frame "---------- Test ----------" {
        # "Template Separator\n(You can make a copy of, or modify, this frame)"
      }
      frame "Test Acquisition Error Handler" {
        # "Test Acquisition Error Handler"
        n126 = call-poly "Enqueue Message.vi"("error in (no error)"=w473, "Message"=w471, "Message Queue"=w472) -> ("error out"=w470:errorcluster)  [unwired: 7 in, 1 out]
      }
      frame "Test Logging Error Handler" {
        # "Test Logging Error Handler"
        n127 = call-poly "Enqueue Message.vi"("error in (no error)"=w481, "Message"=w480, "Message Queue"=w478) -> ("error out"=w479:errorcluster)  [unwired: 7 in, 1 out]
      }
      frame "New Category: 1" {
        # "Your code here.\n(You can make a copy of, or modify, this frame)"
      }
    }
    n128 = call "Error Handler - Message Handling Loop.vi"("element"=w68, "Error Handler Message"="Error Handler" ("Message"), "error in (no error)"=w81, "Message Queue"=w72) -> ("dup error in"=w90:errorcluster)  [unwired: 6 in, 1 out]
  }
  n129 = call "Acquisition Message Loop.vi"("error in (no error)"=w19, "Data Queue"=w8, "Data Notifier"=w10, "Message Queues"=w21) -> ("error out"=w23:errorcluster)  [unwired: 7 in]
  n130 = call "Logging Message Loop.vi"("error in (no error)"=w19, "Data Queue"=w8, "Message Queues"=w21) -> ("error out"=w20:errorcluster)  [unwired: 8 in]
  n131 = while "Data Display Loop" {
    tunnel: w10 -> [w493]
    stop <- w491 stop-if-true
    # "Data Display Loop"
    n132 = Wait on Notification(notifier=w493) -> (notification=→"Data":waveform(dbl)[], error out=w491:errorcluster)  [unwired: 3 in, 2 out]
  }
  n133 = case shown="\"easy copy\"" "DO NOT RUN!!" {
    frame "easy copy" {
      (unwired) "" ("Message")
      # "System_Label"
      n134 = call-poly "Enqueue Message.vi"("Message Queue"=refnum<queue> refnum) -> ()  [unwired: 9 in, 2 out]
    }
    frame Default {
    }
  }
  n135 = Unregister For Events(event registration refnum=w16, error in=w26) -> (error out=w17:errorcluster)
  n136 = case shown="\"easy copy\"" "DO NOT RUN!!" {
    frame Default {
    }
    frame "easy copy" {
      (unwired) "" ("Message")
      # "System_Label"
      n137 = call-poly "Enqueue Message.vi"("Message Queue"=refnum<queue> refnum) -> ()  [unwired: 9 in, 2 out]
    }
  }
  n138 = Merge Errors(w17, w27, w23, w20) -> (w5:errorcluster)
  n139 = call "Destroy User Event - Stop.vi"("error in (no error)"=w5, "User Event - Stop"=w24) -> ("error out"=w7:errorcluster)  [unwired: 9 in]
  n140 = disable-structure shown="RUN_TIME_ENGINE==True" {
    disable-tunnel: w7 -> [_ _]
    frame condition #0 (active) {
    }
    frame condition #1 {
      # "Call Quit LabVIEW if running as a built application."
      n141 = Quit LabVIEW() -> ()  [unwired: 1 in]
    }
  }
